vi "Periodic Tasks.vi"(8 "error in":errorcluster) -> ()   [LabVIEW 2013]
doc: "This VI runs in parallel to other tasks. It can contain as many user-defined periodic loops as you need. These can carry out PID or other sorts of timed response."
uses:
  <vilib>/Rock Robotics/SystemInterfaces/Utilities/FPGA_UtilitiesLED Source.ctl
  <vilib>/Rock Robotics/SystemInterfaces/Utilities/FPGA_UtilitiesLED State.ctl
  <vilib>/Rock Robotics/WPI/Compressor/WPI_CompressorGetSetRefNum.vi
  Robot Global Data.vi
panel:
  out "DIO":bool
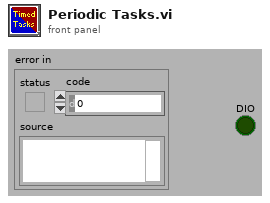
[diagram p1: front panel]
types:
  T1 = typedef "FPGA_UtilitiesLED State.ctl" = enum16{"Off", "On", "Toggle"}
  T2 = typedef "FPGA_UtilitiesLED Source.ctl" = enum16{"User LED", "FPGA LED"}
  T3 = typedef "WPI_MotorControlDeviceRef.ctl" = cluster{"DeviceStatus":errorcluster, "Type":enum16{"PWM", "CAN"}, "PWM":cluster{"Digital Module":T4, "PWM Channel":T5, "DeadBand":T6}, "CAN":cluster{"Device Number":u8, "Control Mode":T7, "Semaphore":T8, "Max Vout":dbl}, "Invert":bool, "TransformRef":T9, "InvTransformRef":T9}
  T4 = typedef "FPGA_TypedefDigitalModule.ctl" = enum16{"Digital Module 1", "Digital Module 2"}
  T5 = typedef "FPGA_DIOPWMChannel.ctl" = enum8{"PWM 1", "PWM 2", "PWM 3", "PWM 4", "PWM 5", "PWM 6", "PWM 7", "PWM 8", "PWM 9", "PWM 10", "Invalid"}
  T6 = typedef "WPI_PWMDeadband.ctl" = cluster{"Name":string, "maxPositivePwm":i32, "minPositivePwm":i32, "centerPwm":i32, "maxNegativePwm":i32, "minNegativePwm":i32, "angularRange":u16}
  T7 = typedef "WPI_CANJaguar_ControlMode.ctl" = enum8{"Percent VBus", "Current", "Speed", "Position", "Voltage"}
  T8 = typedef "Semaphore RefNum" = refnum<k1>
  T9 = typedef "WPI_PWMTransform_ConPane.ctl" = refnum<vi>
  T10 = typedef "WPI_CompressorDevRef.ctl" = cluster{"DevStatus":errorcluster, "DigitalInputDevRef":T11, "RelayDevRef":T13}
  T11 = typedef "WPI_DigitalInputDevRef.ctl" = cluster{"DevStatus":errorcluster, "DIO Channel":T12, "Digital Module":T4}
  T12 = typedef "FPGA_DIOChannel.ctl" = enum8{"DIO 1", "DIO 2", "DIO 3", "DIO 4", "DIO 5", "DIO 6", "DIO 7", "DIO 8", "DIO 9", "DIO 10", "DIO 11", "DIO 12", "DIO 13", "DIO 14", "Invalid"}
  T13 = typedef "WPI_RelayDevRef.ctl" = cluster{"DevStatus":errorcluster, "Relay Channel":T14, "Digital Module":T4, "Relay Direction":T15}
  T14 = typedef "FPGA_DIORelayChannel.ctl" = enum8{"Relay 1", "Relay 2", "Relay 3", "Relay 4", "Relay 5", "Relay 6", "Relay 7", "Relay 8", "Invalid"}
  T15 = typedef "WPI_RelayDirection.ctl" = enum16{"Both directions", "Forward only", "Reverse only"}
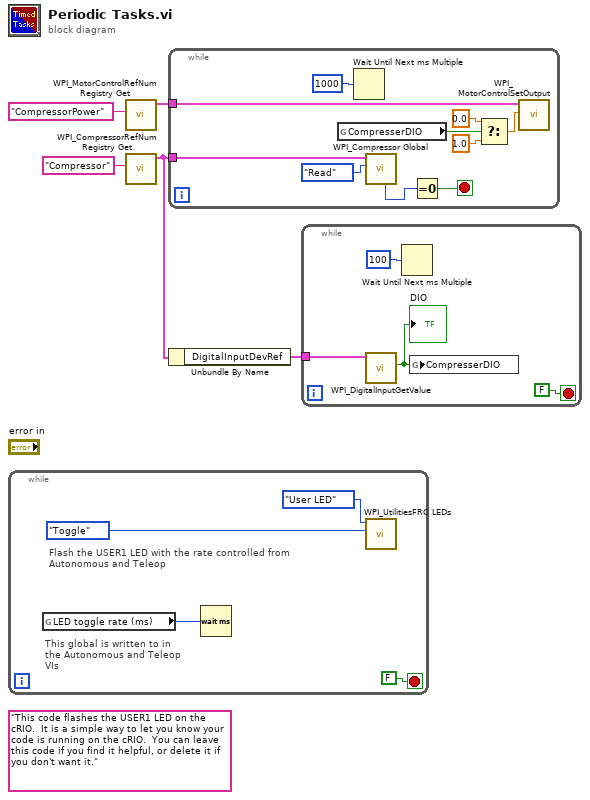
[diagram p0: block diagram]
diagram:
  (unwired) "This code flashes the USER1 LED on the cRIO.  It is a simple way to let you know your code is running on the cRIO.  You can leave this code if you find it helpful, or delete it if you don't want it."
  n1 = while {
    stop <- FALSE stop-if-true
    # "This global is written to in the Autonomous and Teleop VIs"
    # "Flash the USER1 LED with the rate controlled from Autonomous and Teleop"
    n2 = global read "Robot Global Data.vi" "LED toggle rate (ms)"() -> (w6:u32)
    n3 = Wait (ms)(milliseconds to wait=w6) -> ()  [unwired: 1 out]
    n4 = call <vilib>:"WPI_UtilitiesFRC LEDs.vi"("State"=FPGA_UtilitiesLED_State."Toggle", "LED Type"=FPGA_UtilitiesLED_Source."User LED") -> ()  [unwired: 1 in, 9 out]
  }
  n5 = call <vilib>:"WPI_MotorControlRefNum Registry Get.vi"("refnum name"="CompressorPower") -> ("MotorControlDevRef"=w3:T3)  [unwired: 9 in, 1 out]
  n6 = call <vilib>:"WPI_CompressorRefNum Registry Get.vi"("refnum name"="Compressor") -> ("CompressorDevRef"=w2:T10)  [unwired: 9 in, 1 out]
  n7 = while {
    tunnel: w2 -> [w19]
    tunnel: w3 -> [w15]
    stop <- w17 stop-if-true
    n8 = global read "Robot Global Data.vi" "CompresserDIO"() -> (w13:bool)
    n9 = Wait Until Next ms Multiple(millisecond multiple=u32 1000 ("timeout in ms (0)")) -> ()  [unwired: 1 out]
    n10 = call <vilib>:"WPI_Compressor Global.vi"("Operation"=enum16{"Read", "Write", "Add", "Remove"}."Read", "CompressorDevRef"=w19) -> ("Compressor Count"=w18:u8)  [unwired: 8 in, 1 out]
    n11 = Equal To 0?(x=w18) -> (x = 0?=w17:bool)
    n12 = Select(t=0.0 ("Output"), s=w13, f=1.0) -> (s? t:f=w12:dbl)
    n13 = call <vilib>:"WPI_MotorControlSetOutput.vi"("Output"=w12, "MotorControlDevRef"=w15) -> ()  [unwired: 7 in, 3 out]
  }
  n14 = Unbundle By Name(w2) -> ("DigitalInputDevRef"=w1:T11)
  n15 = while {
    tunnel: w1 -> [w21]
    stop <- FALSE stop-if-true
    n16 = call <vilib>:"WPI_DigitalInputGetValue.vi"("DigitalInputDevRef"=w21) -> ("Value"=w20:bool)  [unwired: 1 in, 9 out]
    "DIO" <- w20
    n17 = Wait Until Next ms Multiple(millisecond multiple=u32 100 ("timeout in ms (0)")) -> ()  [unwired: 1 out]
    n18 = global write "Robot Global Data.vi" "CompresserDIO"(w20) -> ()
  }
